vi "__6501_DigitalOut_1line.vi"(0 "OFF,ON(0,1)":i32, 1 "line(0...7)":i32, 2 "Port(0,1,2)":i32, 3 "Dev(1,2..)":i32=1) -> ()   [LabVIEW 2017]
uses:
  <vilib>/Utility/error.llb/DialogType.ctl
  <vilib>/DAQmx/write.llb/DAQmx Write (Digital Bool 1Line 1Point).vi
  <vilib>/DAQmx/create/channels.llb/DAQmx Create Channel (DO-Digital Output).vi
  <vilib>/DAQmx/miscellaneous.llb/DAQmx Fill In Error Info.vi
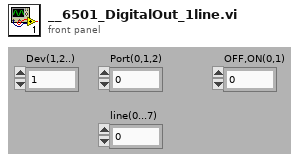
[diagram p1: front panel]
types:
  T1 = typedef "DialogType.ctl" = u16
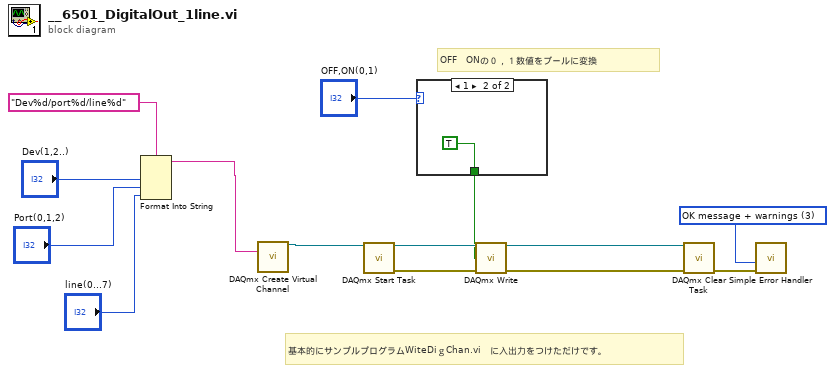
[diagram p0: block diagram]
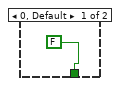
[diagram p2: hidden frame]
diagram:
  w9 = T1 3 items=["no dialog", "OK message", "continue or stop message", "OK message + warnings", "continue/stop + warnings"] ("type of dialog (OK msg:1)")
  # "OFF　ONの０，１数値をブールに変換"
  # "基本的にサンプルプログラムWiteDiｇChan.vi　に入出力をつけただけです。"
  n1 = Format Into String(format string="Dev%d/port%d/line%d" ("文字列"), "Dev(1,2..)", "Port(0,1,2)", "line(0...7)") -> (resulting string=w3:string)  [unwired: 2 in, 1 out]
  n2 = call-poly <vilib>:"DAQmx Create Virtual Channel.vi"("lines"=w3) -> ("task out"=w8:refnum<k21>)  [unwired: 13 in, 1 out]
  n3 = call <vilib>:"DAQmx Start Task.vi"("task/channels in"=w8) -> ("task out"=w11:refnum<k21>, "error out"=w14:errorcluster)  [unwired: 13 in]
  n4 = case shown="1" "OFF,ON(0,1)" {
    tunnel: [FALSE ("ON,OFF") TRUE ("ON,OFF")] -> w1
    frame 0, Default {
    }
    frame 1 {
    }
  }
  n5 = call-poly <vilib>:"DAQmx Write.vi"("task/channels in"=w11, "data"=w1, "error in"=w14) -> ("task out"=w10:refnum<k21>, "error out"=w13:errorcluster)  [unwired: 10 in, 1 out]
  n6 = call <vilib>:"DAQmx Clear Task.vi"("task in"=w10, "error in"=w13) -> ("error out"=w12:errorcluster)  [unwired: 13 in]
  n7 = call <vilib>:"Simple Error Handler.vi"("type of dialog (OK msg:1)"=w9, "error in (no error)"=w12) -> ()  [unwired: 3 in, 5 out]
